vi "WaitForGoodIPAddress.vi"() -> (0 "Good?":bool)   [LabVIEW 2015]
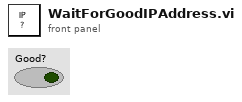
[diagram p1: front panel]
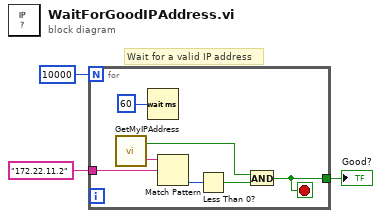
[diagram p0: block diagram]
diagram:
  # "Wait for a valid IP address"
  n1 = for {
    N: 10000 -> [_]
    tunnel: [w5] -> w3
    tunnel: "172.22.11.2" ("IP Address") -> [w8]
    stop <- w5 stop-if-true
    n2 = call "GetMyIPAddress.vi"() -> ("URI"=w9:string, "Good?"=w6:bool)  [unwired: 2 in]
    n3 = Wait (ms)(milliseconds to wait=u32 60) -> ()  [unwired: 1 out]
    n4 = Match Pattern(string=w9, regular expression=w8) -> (offset past match=w7:i32)  [unwired: 1 in, 3 out]
    n5 = Less Than 0?(x=w7) -> (x < 0?=w4:bool)
    n6 = And(x=w6, y=w4) -> (x .and. y?=w5:bool)
  }
  "Good?" <- w3
